vi "Get Name.vi"(8 "error in (no error)":errorcluster, 11 "Dependency Source_Custom in":refnum<class "Dependency Source_GPM.lvclass">) -> (0 "error out":errorcluster, 2 "Dependency Source Name":string, 3 "Dependency Source_Custom out":refnum<class "Dependency Source_GPM.lvclass">)   [LabVIEW 2019, in "Project.Dependencies Finder.lvlib" / "Dependency Source_GPM.lvclass"]
doc: "Return the name of the dependency source. \n\nThis implementation returns 'GPM'."
uses:
  Dependency Source_GPM.lvclass
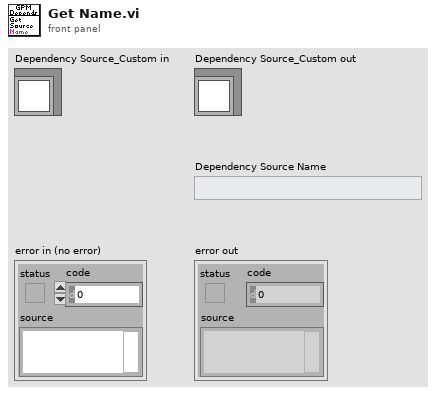
[diagram p1: front panel]
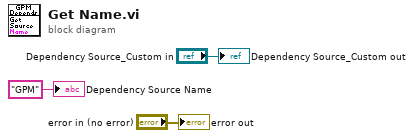
[diagram p0: block diagram]
diagram:
  "error out" <- "error in (no error)"
  "Dependency Source Name" <- "GPM" ("Dependency Source Name")
  "Dependency Source_Custom out" <- "Dependency Source_Custom in"
